vi "fi-display-can-table.vi"(5 "table.ref":refnum<vi>, 8 "error in (no error)":errorcluster, 11 "fi in":refnum<class "frameInput.lvclass">) -> (0 "error out":errorcluster, 3 "fi out":refnum<class "frameInput.lvclass">)   [LabVIEW 2015]
uses:
  frameInput.lvclass
  class.can.table/CAN_table.ctl
  class.can.table/CANtable.lvclass
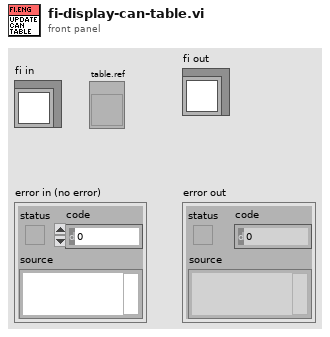
[diagram p1: front panel]
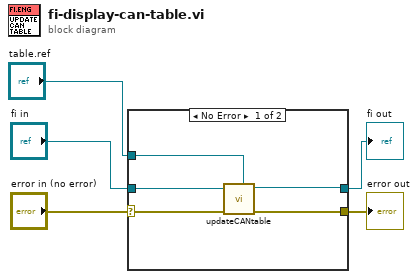
[diagram p0: block diagram]
diagram:
  n1 = case shown="No Error" "error in (no error)" {
    selector: "error in (no error)" -> [w10 w12]
    tunnel: [w9 w12] -> w4
    tunnel: [w6 w11] -> w2
    tunnel: "fi in" -> [w7 w11]
    tunnel: "table.ref" -> [w8 _]
    frame No Error {
      n2 = call "updateCANtable.vi"("table.ref"=w8, "error in (no error)"=w10, "CANtable.lvclass"=w7) -> ("error out"=w9:errorcluster, "CANtable.lvclass 2"=w6:refnum<class "frameInput.lvclass">)  [unwired: 7 in]
    }
    frame Error {
    }
  }
  "error out" <- w4
  "fi out" <- w2
